vi "Calibration.vi"(0 "Mode":T3, 5 "Calib file":path, 9 "Simulate/Run":T2) -> (14 "Calib const":string[][](array[string]), 16 "Coefficients":dbl[][](array[numeric]) format="%.2f", 19 "Status Out":T1)   [LabVIEW 2010]
uses:
  Anemometry Sub Vis/Calibration/Calib_mode.ctl
  Anemometry Sub Vis/Controls/User_Specific_mode.ctl
  Anemometry Sub Vis/Gen Trav/Multi_Run_Status.ctl
  Anemometry Sub Vis/Controls/Post_Process.ctl
  Anemometry Sub Vis/File/Setup_Filetype.ctl
  Anemometry Sub Vis/Controls/Save_Data.ctl
  Anemometry Sub Vis/Controls/Setup.ctl
  Anemometry Sub Vis/Controls/App_Global.ctl
  Anemometry Sub Vis/Globals/Meas_global.vi
  Anemometry Sub Vis/Globals/Calib_global.vi
  Anemometry Sub Vis/Globals/Plug_in_data_global.vi
  Anemometry Sub Vis/Acquisition/PWA/PWAtasksGLOBAL.vi
  <vilib>/Analysis/NI_AALBase.lvlib
panel:
  in  "-ve Ref Values":bool
  out "String":string
  in  "polynomial order":i32=2 min=1 max=3 step=1
  out "Ref velocity":dbl[](array[numeric])=[2.4275346736, 2.4395664609, 2.453235235, 2.4247395837, 2.4277603784, 2.41169823, 2.4254144559, 2.424896502176921] format="%.3f"
  out "labels":string[](array[string])=["XW1 Volt", "XW2 Volt", "Entered Val", "Selector"]
  in  "Point selector 3":cluster{"Y":dbl, "X":dbl, "t/f":bool}[](array[cluster]) {"X" format="%#.2g"; "Y" format="%#.3f"}
  in  "n":dbl=0.45 format="%.4f"
  in  "Fixed n":bool=TRUE
  out "Sample of input signals":dbl[][](graph)
  in  "Sampling speeds":T4={"Samples /ch"=600, "Sampling Rate /ch (Hz)"=100.0} {"Sampling Rate /ch (Hz)" min=0 format="%.2f"; "Samples /ch" min=0 step=1}
  out "Calibration plot":cluster{cluster{dbl, dbl}[]}[](graph)
  in  "Point selector 4":T5(array[cluster]) {"Y2" format="%#.2f"; "X" format="%#.3f"; "Y" format="%#.2f"}
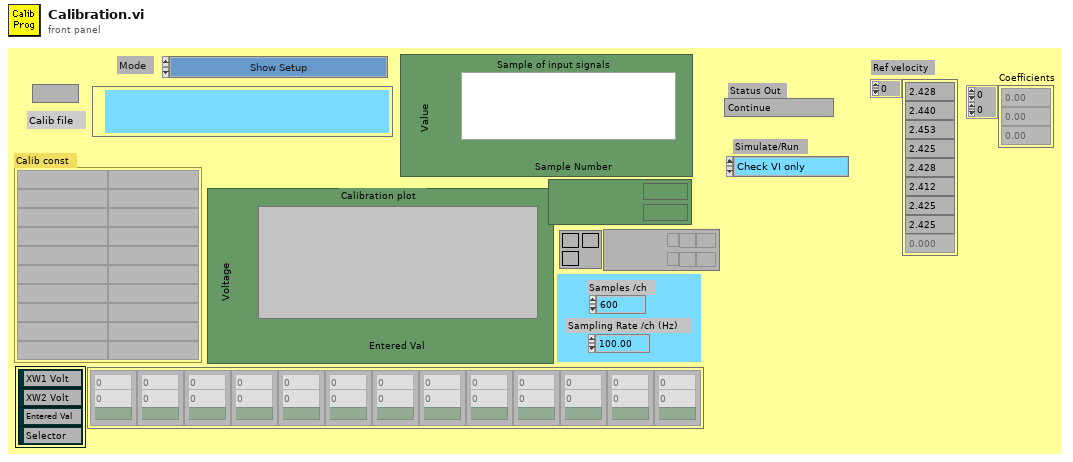
[diagram p1: front panel]
types:
  T1 = typedef "Multi_Run_Status.ctl" = enum16{"Continue", "Jump to Next Point", "Jump to Next Row", "Jump To Fall Back", "Terminate Run"}
  T2 = typedef "User_Specific_mode.ctl" = enum16{"Check VI only", "Run VI"}
  T3 = typedef "Calib_mode.ctl" = enum16{"Show Setup", "Take a New Calibration Point", "Refit Curve", "Setup Front Panel"}
  T4 = cluster{"Samples /ch":i32, "Sampling Rate /ch (Hz)":sgl}
  T5 = cluster{"Y":dbl, "Y2":dbl, "X":dbl, "t/f":bool}[]
  T6 = typedef "Post_Process.ctl" = enum16{"Take New Data", "Post Process Raw Data File"}
  T7 = typedef "Setup_Filetype.ctl" = enum16{"Measurement Setups", "Calibration Setups", "General", "Results File Plotter Setups", "Speed Calib Tweaks"}
  T8 = typedef "Save_Data.ctl" = enum16{"Save No Data", "Save Data"}
  T9 = typedef "Setup.ctl" = enum16{"Run Program", "Show Setup", "Save Current Setup", "Setup Front Panel"}
  T10 = typedef "App_Global.ctl" = enum16{"Read Global", "Write to Global", "Initialise Array"}
  T11 = enum32{"existing file", "new file", "new or existing file", "existing dir", "new dir", "new or existing dir", "existing file (use LLBs)", "new file (use LLBs)", "new or existing file (use LLBs)", "new or existing file or directory (use LLBs)"}
  T12 = typedef "Cal_Inst_type.ctl" = enum16{"Propeller anemometer", "Pressure Transducer", "Hot wire", "Cross wire velocity", "Cross wire angle", "Generic Linear", "Generic Polynomial", "Generic BackPoly", "Fast FID", "Thermocouple", "Cold wire", "Pulsed Wire"}
  T13 = typedef "Ref_Inst_type.ctl" = enum16{"Propellor anemometer", "Pressure Transducer", "Raw voltage", "Pitot-static tube", "Preston tube", "Generic Linear", "Generic Polynomial", "Thermocouple", "LDA", "Enter Value", "ADAM Channel"}
  T14 = cluster{"2nd Ref type":T13, "2nd inst present":bool}
  T15 = typedef "Velocity_cluster.ctl" = cluster{"Name":string, "U":dbl, "u^2":dbl, "u^3/(u^2)^(1.5)":dbl, "u^4/(u^2)^2 -3":dbl, "% u'/U":dbl, "Mean % Err":dbl, "u^4":dbl}
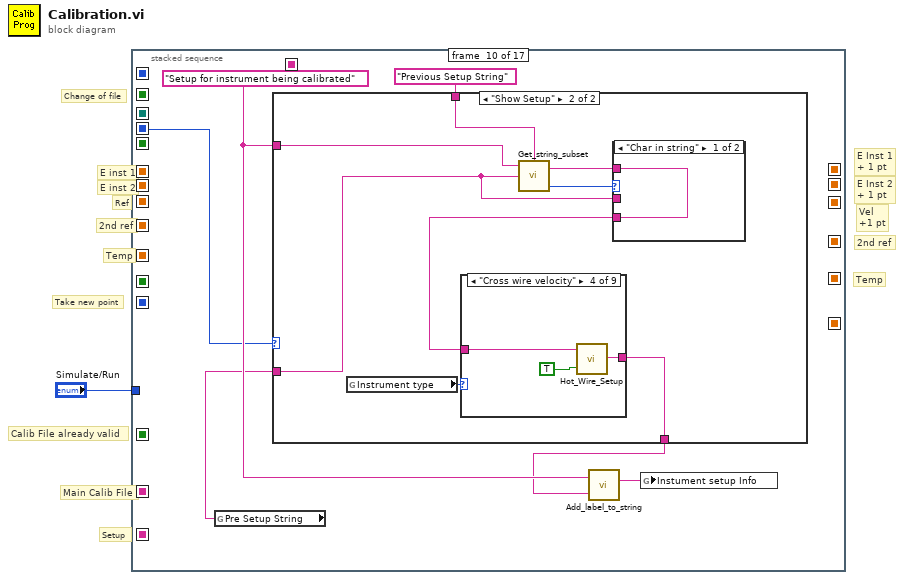
[diagram p0: block diagram]
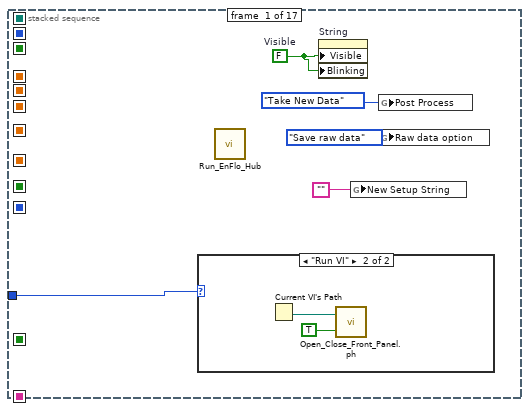
[diagram p2: hidden frame]
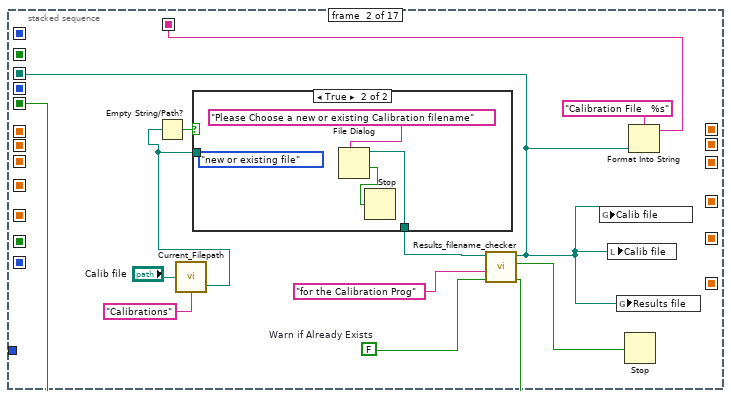
[diagram p4: hidden frame]
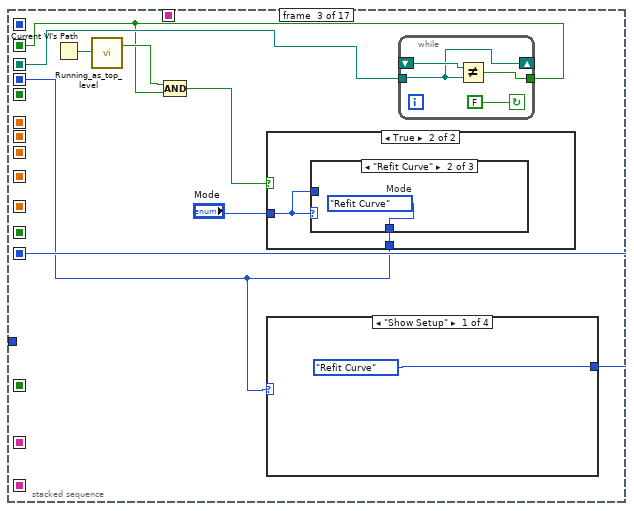
[diagram p6: hidden frame]
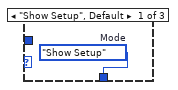
[diagram p8: hidden frame]
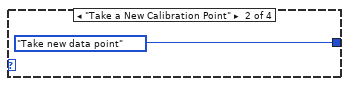
[diagram p10: hidden frame]
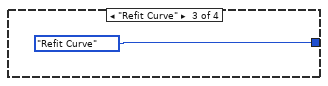
[diagram p11: hidden frame]
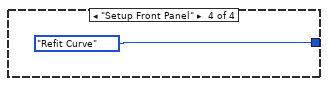
[diagram p12: hidden frame]
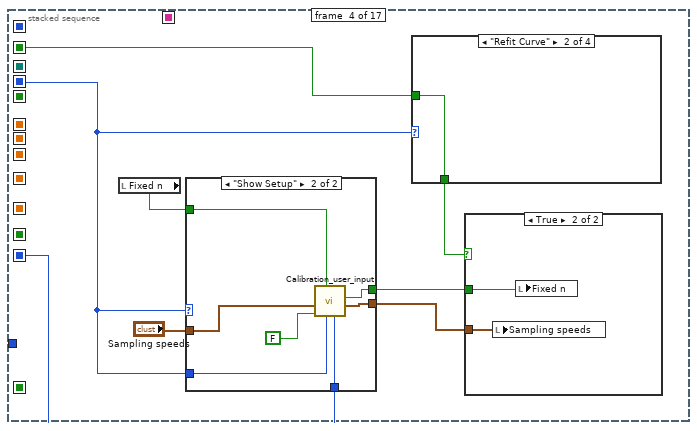
[diagram p13: hidden frame]
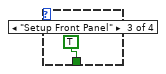
[diagram p15: hidden frame]
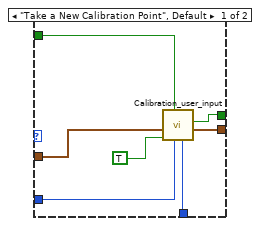
[diagram p18: hidden frame]
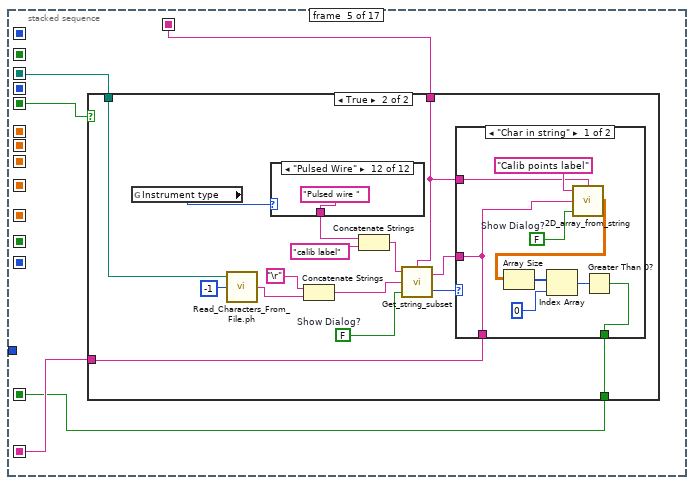
[diagram p19: hidden frame]
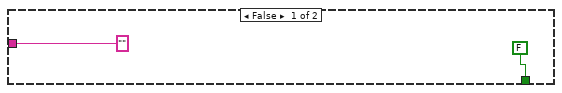
[diagram p20: hidden frame]
diagram:
  # "Change of file"
  # "Take new point"
  # "Calib File already valid"
  # "Main Calib File"
  # "Temp"
  # "Temp"
  # "Setup"
  # "E inst 1"
  # "Ref"
  # "E Inst 1\n+ 1 pt"
  # "Vel\n+1 pt"
  # "E inst 2"
  # "E Inst 2\n+ 1 pt"
  # "2nd ref"
  # "2nd ref"
  n1 = stacked-sequence {
    seq-local: [_ _ _ _ _ _ _ _ _ _ _ w489 _ _ _ _ _] -> [_ _ _ _ _ _ _ _ _ _ _ _ w674 _ _ _ _]
    seq-local: [_ _ _ _ _ _ _ _ _ _ _ w488 _ _ _ _ _] -> [_ _ _ _ _ _ _ _ _ _ _ _ w677 _ _ w740 _]
    seq-local: [_ _ _ _ _ _ _ w376 _ _ _ _ _ _ _ _ _] -> [_ _ _ _ _ _ _ _ _ _ _ w491 _ _ _ _ _]
    seq-local: [_ _ _ _ _ _ _ w375 _ _ _ _ _ _ _ _ _] -> [_ _ _ _ _ _ _ _ _ _ _ w490 _ _ _ _ _]
    seq-local: [_ _ _ _ _ _ _ w374 _ _ _ _ _ _ _ _ _] -> [_ _ _ _ _ _ _ _ _ _ _ w486 _ _ _ _ _]
    seq-local: [_ _ _ _ _ _ _ _ _ _ _ w487 _ _ _ _ _] -> [_ _ _ _ _ _ _ _ _ _ _ _ w676 _ _ _ _]
    seq-local: [_ _ _ _ _ _ _ w373 _ _ _ _ _ _ _ _ _] -> [_ _ _ _ _ _ _ _ _ _ _ w485 _ _ _ _ _]
    seq-local: [_ _ _ _ _ _ _ _ _ _ _ w484 _ _ _ _ _] -> [_ _ _ _ _ _ _ _ _ _ _ _ w671 _ _ _ _]
    seq-local: [_ _ _ _ w78 _ _ _ _ _ _ _ _ _ _ _ _] -> [_ _ _ _ _ _ _ w362 _ _ _ _ _ _ _ _ _]
    seq-local: [_ _ _ _ w79 _ _ _ _ _ _ _ _ _ _ _ _] -> [_ _ _ _ _ _ _ w363 _ _ _ _ _ _ _ _ _]
    seq-local: [_ _ _ _ _ _ _ _ _ _ w464 _ _ _ _ _ _] -> [_ _ _ _ _ _ _ _ _ _ _ _ _ _ w718 _ _]
    seq-local: [_ _ _ _ _ _ _ _ _ _ _ w482 _ _ _ _ _] -> [_ _ _ _ _ _ _ _ _ _ _ _ w675 _ _ _ _]
    seq-local: [_ _ _ _ _ _ _ w372 _ _ _ _ _ _ _ _ _] -> [_ _ _ _ _ _ _ _ _ _ _ w481 _ _ _ _ _]
    seq-local: [_ w13 _ _ _ _ _ _ _ _ _ _ _ _ _ _ _] -> [_ _ w29 _ w77 _ _ _ _ _ w465 w479 _ w700 w727 w741 _]
    seq-local: [_ w18 _ _ _ _ _ _ _ _ _ _ _ _ _ _ _] -> [_ _ _ _ w76 _ _ _ w405 _ _ _ _ _ _ _ _]
    seq-local: [_ _ w32 _ _ _ _ _ _ _ _ _ _ _ _ _ _] -> [_ _ _ w50 _ _ _ _ _ _ _ w478 _ _ _ w742 _]
    seq-local: [_ _ w25 _ _ _ _ _ _ _ _ _ _ _ _ _ _] -> [_ _ _ w49 _ _ _ _ _ w422 _ _ _ _ _ _ w786]
    seq-local: [_ _ _ _ _ _ _ w364 _ _ _ _ _ _ _ _ _] -> [_ _ _ _ _ _ _ _ w403 _ _ _ _ _ _ _ _]
    seq-local: [_ _ _ _ _ _ _ _ _ _ _ _ w672 _ _ _ _] -> [_ _ _ _ _ _ _ _ _ _ _ _ _ w684 _ _ _]
    seq-local: [_ _ _ _ _ _ _ _ _ _ _ _ w670 _ _ _ _] -> [_ _ _ _ _ _ _ _ _ _ _ _ _ w699 _ _ _]
    seq-local: [_ _ w28 _ _ _ _ _ _ _ _ _ _ _ _ _ _] -> [_ _ _ w47 _ _ _ _ w402 _ _ _ _ _ _ _ _]
    seq-local: [_ w12 _ _ _ _ _ _ _ _ _ _ _ _ _ _ _] -> [_ _ _ _ w75 _ _ w357 _ _ _ _ _ _ _ _ _]
    tunnel: "Simulate/Run" -> [w5 _ _ _ _ _ _ _ _ _ _ _ _ _ _ _ _]
    frame #0 {
      w3 = FALSE  # Visible
      n2 = case shown="\"Run VI\"" w5 {
        frame "Check VI only" {
        }
        frame "Run VI" {
          n3 = Current VI's Path() -> (path=w7:path)
          n4 = call "Open_Close_Front_Panel.ph.vi"("Front Panel Window:Open"=TRUE, "VI path"=w7) -> ()  [unwired: 2 out]
        }
      }
      n5 = call "Run_EnFlo_Hub.vi"() -> ()  [unwired: 8 out]
      n6 = property on="String" class="Str"("Visible"=w3, "Blinking"=w3) -> ()  [unwired: 2 in, 2 out]
      n7 = global write "Calib_global.vi" "New Setup String"("") -> ()
      n8 = global write "Meas_global.vi" "Post Process"(Post_Process."Take New Data" ("Post Process")) -> ()
      n9 = global write "Meas_global.vi" "Raw data option"(enum16{"Save raw data", "Raw data not saved"}."Save raw data" ("Raw data option")) -> ()
    }
    frame #1 {
      w19 = FALSE  # Warn if Already Exists
      n10 = call "Current_Filepath.vi"("Filename in"="Calib file", "Data Type"="Calibrations") -> ("Filename Out"=w10:path)  [unwired: 1 out]
      n11 = Empty String/Path?(string/path=w10) -> (empty?=w15:bool)
      n12 = case shown="True" w15 {
        tunnel: w10 -> [w21 _]
        tunnel: [w21 w23] -> w17
        frame False {
        }
        frame True {
          (unwired) T11."new or existing file" ("select mode (2)")
          n13 = File Dialog(7:"Please Choose a new or existing Calibration filename" ("Promp if not found")) -> (1:w22:bool, 3:w23:path)  [unwired: 1 in, 7 out]
          n14 = Stop(stop? (T)=w22) -> ()
        }
      }
      n15 = call "Results_filename_checker.vi"("Warn if Already Exists"=w19, "Comment"="for the Calibration Prog", "Results file"=w17) -> ("exists?"=w18:bool, "cancelled"=w16:bool, "Results file output"=w13:path)  [unwired: 2 in, 1 out]
      n16 = global write "Calib_global.vi" "Calib file"(w13) -> ()
      n17 = local write "Calib file"(w13) -> ()
      n18 = global write "Meas_global.vi" "Results file"(w13) -> ()
      n19 = Stop(stop? (T)=w16) -> ()
      n20 = Format Into String(format string="Calibration File   %s", w13) -> (resulting string=w12:string)  [unwired: 2 in, 1 out]
    }
    frame #2 {
      n21 = Current VI's Path() -> (path=w31:path)
      n22 = call "Running_as_top_level.vi"("Vi path name"=w31) -> ("Top Level"=w30:bool)  [unwired: 1 out]
      n23 = while {
        shift-right: [w41] -> _
        shift-left: _ -> [w42]
        tunnel: w29 -> [w41]
        tunnel: [w40] -> w28
        stop <- FALSE continue-if-true
        n24 = Not Equal?(x=w42, y=w41) -> (x != y?=w40:bool)
      }
      n25 = Compound Arithmetic op=AND(w30, w28) -> (w27:bool)
      n26 = case shown="True" w27 {
        tunnel: "Mode" -> [w33 w34]
        tunnel: [w33 w35] -> w25
        frame False {
        }
        frame True {
          n27 = case shown="\"Refit Curve\"" w34 {
            tunnel: [w36 w37 w38] -> w35
            tunnel: w34 -> [_ _ w38]
            frame "Show Setup", Default {
              w36 = Calib_mode."Show Setup"  # Mode
            }
            frame "Refit Curve" {
              w37 = Calib_mode."Refit Curve"  # Mode
            }
            frame "Setup Front Panel" {
            }
          }
        }
      }
      n28 = case shown="\"Show Setup\"" w25 {
        tunnel: [enum16{"Take new data point", "Refit Curve"}."Refit Curve" ("data mode") enum16{"Take new data point", "Refit Curve"}."Take new data point" ("data mode") enum16{"Take new data point", "Refit Curve"}."Refit Curve" ("data mode") enum16{"Take new data point", "Refit Curve"}."Refit Curve" ("data mode")] -> w32
        frame "Show Setup" {
        }
        frame "Take a New Calibration Point" {
        }
        frame "Refit Curve" {
        }
        frame "Setup Front Panel" {
        }
      }
    }
    frame #3 {
      n29 = local read "Fixed n"() -> (w52:bool)
      n30 = case shown="\"Show Setup\"" w49 {
        tunnel: "Sampling speeds" -> [w67 w74]
        tunnel: w49 -> [w65 w72]
        tunnel: w50 -> [w64 w71]
        tunnel: [w63 w70] -> w53
        tunnel: w52 -> [w61 w69]
        tunnel: [w62 w68] -> w51
        frame "Take a New Calibration Point", Default {
          n31 = call "Calibration_user_input.vi"("data mode"=w64, "Mode"=w65, "Fixed n"=w61, "OK"=TRUE, "Sampling speeds"=w67) -> ("Sampling speeds Output"=w63:T4, "Fixed n out"=w62:bool)  [unwired: 2 in, 3 out]
        }
        frame "Show Setup" {
          n32 = call "Calibration_user_input.vi"("data mode"=w71, "Mode"=w72, "Fixed n"=w69, "OK"=FALSE, "Sampling speeds"=w74) -> ("Sampling speeds Output"=w70:T4, "Fixed n out"=w68:bool)  [unwired: 5 out]
        }
      }
      n33 = case shown="\"Refit Curve\"" w49 {
        tunnel: [w55 w56 TRUE w58] -> w48
        tunnel: w47 -> [w55 w56 _ w58]
        frame "Show Setup" {
        }
        frame "Refit Curve" {
        }
        frame "Setup Front Panel" {
        }
        frame "Take a New Calibration Point" {
        }
      }
      n34 = case shown="True" w48 {
        tunnel: w53 -> [_ w60]
        tunnel: w51 -> [_ w59]
        frame False {
        }
        frame True {
          n35 = local write "Sampling speeds"(w60) -> ()
          n36 = local write "Fixed n"(w59) -> ()
        }
      }
    }
    frame #4 {
      n37 = case shown="True" w76 {
        tunnel: ["" ("Output string") w96] -> w79
        tunnel: [FALSE w95] -> w78
        tunnel: w77 -> [_ w87]
        tunnel: w75 -> [_ w82]
        frame False {
        }
        frame True {
          w86 = FALSE  # Show Dialog?
          n38 = global read "Calib_global.vi" "Instrument type"() -> (w90:T12)
          n39 = call "Read_Characters_From_File.ph.vi"("file path (dialog if empty)"=w87, "number of characters (all:-1)"=-1) -> ("character string"=w84:string)  [unwired: 7 out]
          n40 = case shown="\"Pulsed Wire\"" w90 {
            tunnel: ["Prop " "Mano " "HW " "Cross wire velocity " "Cross wire angle " "Generic Inst " "Generic Polynomial " "Generic BackPoly " "Fast FID " "Thermocouple " "Cold wire " "Pulsed wire "] -> w91
            frame "Propeller anemometer" {
            }
            frame "Pressure Transducer" {
            }
            frame "Hot wire" {
            }
            frame "Cross wire velocity" {
            }
            frame "Cross wire angle" {
            }
            frame "Generic Linear" {
            }
            frame "Generic Polynomial" {
            }
            frame "Generic BackPoly" {
            }
            frame "Fast FID" {
            }
            frame "Thermocouple" {
            }
            frame "Cold wire" {
            }
            frame "Pulsed Wire" {
            }
          }
          n41 = Concatenate Strings("\r", w84) -> (w83:string)
          n42 = Concatenate Strings(w91, "calib label") -> (w92:string)
          n43 = call "Get_string_subset.vi"("String Name"=w82, "Show Dialog?"=w86, "String to split"=w83, "File Label"=w92) -> ("Status"=w89:enum16{"Char in string", "Char not in string"}, "Output string"=w88:string)
          n44 = case shown="\"Char in string\"" w89 {
            tunnel: w88 -> [w115 _]
            tunnel: [w115 ""] -> w96
            tunnel: [w110 FALSE] -> w95
            tunnel: w82 -> [w109 _]
            frame "Char in string" {
              w116 = FALSE  # Show Dialog?
              n45 = call "2D_array_from_string.vi"("String Name"=w109, "Show Dialog?"=w116, "Input string"=w115, "Array title"="Calib points label") -> ("2D data array"=w114:dbl[][])
              n46 = Array Size(array=w114) -> (size(s)=w113:i32[])
              n47 = Index Array(array=w113, index=0 ("Index")) -> (element=w111:i32)
              n48 = Greater Than 0?(x=w111) -> (x > 0?=w110:bool)
            }
            frame "Char not in string" {
            }
          }
        }
      }
    }
    frame #5 {
      w122 = ""
      n49 = global read "Calib_global.vi" "2nd ref instrument"() -> (w129:T14)
      n50 = global read "Calib_global.vi" "Ref Instrument type"() -> (w130:T13)
      n51 = Unbundle By Name(w129) -> ("2nd Ref type"=w127:T13, "2nd inst present"=w128:bool)
      n52 = global read "Calib_global.vi" "Instrument type"() -> (w133:T12)
      n53 = case shown="\"Propellor anemometer\"" w130 {
        tunnel: [w159 w162 w166 w168 w171 w174 w177 w180 w183 string[] [] string[] []] -> w126
        tunnel: [FALSE FALSE FALSE FALSE TRUE FALSE FALSE FALSE FALSE FALSE FALSE] -> w121
        frame "Propellor anemometer" {
          n54 = Build Array("Prop Velocity") -> (w159:string[])
        }
        frame "Pressure Transducer" {
          n55 = Build Array("Pressure Trans") -> (w162:string[])
        }
        frame "Raw voltage" {
          n56 = Build Array("Raw Voltage") -> (w166:string[])
        }
        frame "Pitot-static tube" {
          n57 = Build Array("Pitot Vel") -> (w168:string[])
        }
        frame "Preston tube" {
          n58 = Build Array("Shear stress") -> (w171:string[])
        }
        frame "Generic Linear" {
          n59 = Build Array("Gen Lin") -> (w174:string[])
        }
        frame "Generic Polynomial" {
          n60 = Build Array("Gen Poly") -> (w177:string[])
        }
        frame "Thermocouple" {
          n61 = Build Array("Thermo") -> (w180:string[])
        }
        frame "LDA" {
          n62 = Build Array("LDA Vel") -> (w183:string[])
        }
        frame "Enter Value" {
        }
        frame "ADAM Channel" {
        }
      }
      n63 = case shown="True" w128 {
        tunnel: w127 -> [_ w136]
        tunnel: [w135 w137] -> w124
        tunnel: w126 -> [w135 _]
        frame False {
        }
        frame True {
          n64 = case shown="\"Propellor anemometer\"" w136 {
            tunnel: [w138 w140 w143 w144 w146 w148 w150 w152 w154 string[] [] string[] []] -> w137
            frame "Propellor anemometer" {
              n65 = Build Array("Prop Velocity") -> (w138:string[])
            }
            frame "Pressure Transducer" {
              n66 = Build Array("Pressure Trans") -> (w140:string[])
            }
            frame "Raw voltage" {
              n67 = Build Array("Raw Voltage") -> (w143:string[])
            }
            frame "Pitot-static tube" {
              n68 = Build Array("Pitot Vel") -> (w144:string[])
            }
            frame "Preston tube" {
              n69 = Build Array("Shear stress") -> (w146:string[])
            }
            frame "Generic Linear" {
              n70 = Build Array("Gen Lin") -> (w148:string[])
            }
            frame "Generic Polynomial" {
              n71 = Build Array("Gen Poly") -> (w150:string[])
            }
            frame "Thermocouple" {
              n72 = Build Array("Thermo") -> (w152:string[])
            }
            frame "LDA" {
              n73 = Build Array("LDA Vel") -> (w154:string[])
            }
            frame "Enter Value" {
            }
            frame "ADAM Channel" {
            }
          }
        }
      }
      n74 = case shown="\"Pulsed Wire\"" w133 {
        tunnel: [w193 w197 w201 w205 w210 w215 w219 w223 w227 w231 w235 w240] -> w123
        tunnel: [FALSE FALSE FALSE FALSE FALSE FALSE TRUE TRUE FALSE FALSE TRUE TRUE] -> w125
        tunnel: [w191 w195 w199 w203 w208 w213 w217 w221 w225 w229 w233 FALSE] -> w120
        tunnel: w121 -> [w191 w195 w199 w203 w208 w213 w217 w221 w225 w229 w233 _]
        frame "Propeller anemometer" {
          n75 = Build Array("Prop Voltage") -> (w193:string[])
        }
        frame "Pressure Transducer" {
          n76 = Build Array("Pressure Trans") -> (w197:string[])
        }
        frame "Hot wire" {
          n77 = Build Array("HW Voltage") -> (w201:string[])
        }
        frame "Cross wire velocity" {
          n78 = Build Array("XW1 Voltage", "XW2 Voltage") -> (w205:string[])
        }
        frame "Cross wire angle" {
          n79 = Build Array("XW1 Voltage", "XW2 Voltage") -> (w210:string[])
        }
        frame "Generic Linear" {
          n80 = Build Array("Generic Voltage") -> (w215:string[])
        }
        frame "Generic Polynomial" {
          n81 = Build Array("Generic Voltage") -> (w219:string[])
        }
        frame "Generic BackPoly" {
          n82 = Build Array("Generic Voltage") -> (w223:string[])
        }
        frame "Fast FID" {
          n83 = Build Array("FF Voltage") -> (w227:string[])
        }
        frame "Thermocouple" {
          n84 = Build Array("Thermo Voltage") -> (w231:string[])
        }
        frame "Cold wire" {
          n85 = Build Array("CW Voltage") -> (w235:string[])
        }
        frame "Pulsed Wire" {
          n86 = local write "polynomial order"(3 ("polynomial order")) -> ()
          n87 = Build Array("PWA 1/TOF") -> (w240:string[])
        }
      }
      n88 = property on="polynomial order" class="DigNum (strict)"("Visible"=w125) -> ()  [unwired: 2 in, 2 out]
      n89 = Build Array (concatenate)(w124, w123, w122, w122, w122) -> (w131:string[])
      n90 = for {
        N: 3 -> [_]
        tunnel: w131 -> [w189] mode=indexing
        i -> [w190]
        n91 = property on="Sample of input signals" class="WFGraph (strict)"("Active Plot"=w190, "Plot.Plot Name"=w189) -> ()  [unwired: 2 in, 2 out]
      }
      n92 = case shown="False" w120 {
        frame False {
          n93 = local write "-ve Ref Values"(FALSE ("-ve Ref Values")) -> ()
        }
        frame True {
        }
      }
      n94 = property on="-ve Ref Values" class="Bool (strict)"("Visible"=w120) -> ()  [unwired: 2 in, 2 out]
    }
    frame #6 {
      n95 = global read "Calib_global.vi" "Instrument type"() -> (w245:T12)
      n96 = global read "Calib_global.vi" "Ref Instrument type"() -> (w244:T13)
      n97 = case shown="\"Propellor anemometer\"" w244 {
        tunnel: ["Prop Vel" "Pressure" "Voltage" "Pitot Vel" "Shear stress" "Generic Linear" "Generic Poly" "Thermo T" "LDA Vel" "Entered Val" "ADAM Channel"] -> w247
        frame "Propellor anemometer" {
        }
        frame "Pressure Transducer" {
        }
        frame "Raw voltage" {
        }
        frame "Pitot-static tube" {
        }
        frame "Preston tube" {
        }
        frame "Generic Linear" {
        }
        frame "Generic Polynomial" {
        }
        frame "Thermocouple" {
        }
        frame "LDA" {
        }
        frame "Enter Value" {
        }
        frame "ADAM Channel" {
        }
      }
      n98 = case shown="\"Pulsed Wire\"" w245 {
        tunnel: [FALSE FALSE TRUE TRUE TRUE FALSE FALSE FALSE FALSE FALSE FALSE FALSE] -> w250
        tunnel: [TRUE TRUE TRUE FALSE FALSE TRUE TRUE TRUE TRUE TRUE TRUE TRUE] -> w249
        tunnel: [FALSE FALSE FALSE TRUE TRUE FALSE FALSE FALSE FALSE FALSE FALSE FALSE] -> w248
        tunnel: w247 -> [w263 w270 w279 w289 w299 w309 w315 w322 w329 w337 w343 w350]
        tunnel: [w266 w273 w282 w292 w302 w311 w318 w325 w332 w339 w346 w353] -> w246
        tunnel: "Selector" -> [w265 w272 w281 w291 w301 w308 w317 w324 w331 w336 w345 w352]
        tunnel: [w264 w271 "E^2" "XW Volt^2" "Y" w310 w315 w323 w329 w338 w343 w350] -> w242
        tunnel: [w263 w270 w277 w287 "X" w309 w316 w322 w330 w337 w344 w351] -> w243
        frame "Propeller anemometer" {
          w264 = "Prop Volt"
          n99 = Build Array(w264, w263, w265) -> (w266:string[])
        }
        frame "Pressure Transducer" {
          w271 = "Voltage"
          n100 = Build Array(w271, w270, w272) -> (w273:string[])
        }
        frame "Hot wire" {
          n101 = Build Array("HW Volt", w279, w281) -> (w282:string[])
          n102 = Concatenate Strings(w279, "^n") -> (w277:string)
        }
        frame "Cross wire velocity" {
          n103 = Build Array("XW1 Volt", "XW2 Volt", w289, w291) -> (w292:string[])
          n104 = Concatenate Strings(w289, "^n") -> (w287:string)
        }
        frame "Cross wire angle" {
          n105 = Build Array("XW1 Volt", "XW2 Volt", w299, w301) -> (w302:string[])
        }
        frame "Generic Linear" {
          w310 = "Gen Volt"
          n106 = Build Array(w310, w309, w308) -> (w311:string[])
        }
        frame "Generic Polynomial" {
          w316 = "Gen Volt"
          n107 = Build Array(w316, w315, w317) -> (w318:string[])
        }
        frame "Generic BackPoly" {
          w323 = "Gen Volt"
          n108 = Build Array(w322, w323, w324) -> (w325:string[])
        }
        frame "Fast FID" {
          w330 = "FF Volt"
          n109 = Build Array(w330, w329, w331) -> (w332:string[])
        }
        frame "Thermocouple" {
          w338 = "Thermo Volt"
          n110 = Build Array(w338, w337, w336) -> (w339:string[])
        }
        frame "Cold wire" {
          w344 = "CW Volt"
          n111 = Build Array(w344, w343, w345) -> (w346:string[])
        }
        frame "Pulsed Wire" {
          w351 = "1/TOF"
          n112 = Build Array(w351, w350, w352) -> (w353:string[])
        }
      }
      "labels" <- w246
      n113 = property on="n" class="DigNum (strict)"("Visible"=w250) -> ()  [unwired: 2 in, 2 out]
      n114 = property on="Fixed n" class="Bool (strict)"("Visible"=w250) -> ()  [unwired: 2 in, 2 out]
      n115 = property on="Calibration plot" class="XYGraph (strict)"("X Scale.Name Label.Text"=w243, "Y Scale.Name Label.Text"=w242) -> ()  [unwired: 2 in, 2 out]
      n116 = property on="Point selector 3" class="Arr (strict)"("Visible"=w249) -> ()  [unwired: 2 in, 2 out]
      n117 = property on="Point selector 4" class="Arr (strict)"("Visible"=w248) -> ()  [unwired: 2 in, 2 out]
    }
    frame #7 {
      # "Case structure to read previous calibration points if required"
      n118 = global read "Calib_global.vi" "Calibration Points"() -> (w361:dbl[])
      n119 = case shown="True" w362 {
        tunnel: w363 -> [_ w396]
        tunnel: [w388 w393] -> w360
        tunnel: w361 -> [w389 w392]
        tunnel: w357 -> [_ w390]
        frame False {
          n120 = Build Array(w389) -> (w388:dbl[][])
        }
        frame True {
          w395 = FALSE  # Show Dialog?
          n121 = Array Size(array=w392) -> (size(s)=w391:i32)
          n122 = call "2D_array_from_string.vi"("String Name"=w390, "Show Dialog?"=w395, "Input string"=w396, "Array title"="Calib points label") -> ("2D data array"=w394:dbl[][])
          n123 = case shown="0" w391 {
            tunnel: w394 -> [w398 w401]
            tunnel: [w398 w400] -> w393
            tunnel: w392 -> [_ w399]
            frame 0 {
            }
            frame 1, Default {
              n124 = Build Array (concatenate)(w401, w399) -> (w400:dbl[][])
            }
          }
        }
      }
      n125 = for {
        tunnel: w360 -> [w378] mode=indexing
        shift-right: [w377] -> w358
        shift-left: dbl[][] [] -> [w379]
        n126 = Array Subset(array=w378, length=2) -> (w382:dbl[])  [unwired: 1 in]
        n127 = Not A Number/Path/Refnum?(number/path/refnum=w382) -> (NaN/Path/Refnum?=w381:bool[])
        n128 = Or Array Elements(Boolean array=w381) -> (logical OR=w380:bool)
        n129 = case shown="False" w380 {
          tunnel: w379 -> [w386 w387]
          tunnel: w378 -> [w385 _]
          tunnel: [w384 w387] -> w377
          frame False {
            n130 = Build Array (concatenate)(w386, w385) -> (w384:dbl[][])
          }
          frame True {
          }
        }
      }
      n131 = Index Array(array=w358, index (col)=0) -> (element=w375:dbl[])  [unwired: 1 in]
      n132 = Index Array(array=w358, index (col)=1) -> (element=w376:dbl[])  [unwired: 1 in]
      n133 = Index Array(array=w358, index (col)=2) -> (element=w374:dbl[])  [unwired: 1 in]
      n134 = Index Array(array=w358, index (col)=3) -> (element=w373:dbl[])  [unwired: 1 in]
      n135 = Index Array(array=w358, index (col)=4) -> (element=w372:dbl[])  [unwired: 1 in]
      n136 = Index Array(array=w358, index (col)=5) -> (element=w365:dbl[])  [unwired: 1 in]
      n137 = Not A Number/Path/Refnum?(number/path/refnum=w365) -> (NaN/Path/Refnum?=w364:bool[])
    }
    frame #8 {
      n138 = And(x=w402, y=w405) -> (x .and. y?=w404:bool)
      n139 = case shown="True" w404 {
        tunnel: w403 -> [_ w406]
        frame False {
        }
        frame True {
          n140 = local read "Point selector 3"() -> (w410:cluster{"Y":dbl, "X":dbl, "t/f":bool}[])
          n141 = local read "Point selector 4"() -> (w407:T5)
          n142 = for {
            tunnel: w410 -> [w418]
            tunnel: [w420] -> w409 mode=indexing
            tunnel: w406 -> [w419] mode=indexing
            i -> [w417]
            n143 = Index Array(array=w418, index=w417) -> (element=w416:cluster{"Y":dbl, "X":dbl, "t/f":bool})
            n144 = Bundle By Name(cluster=w416, "t/f"=w419) -> (w420:cluster{"Y":dbl, "X":dbl, "t/f":bool})
          }
          n145 = for {
            tunnel: w407 -> [w413]
            tunnel: [w415] -> w408 mode=indexing
            tunnel: w406 -> [w414] mode=indexing
            i -> [w412]
            n146 = Index Array(array=w413, index=w412) -> (element=w411:cluster{"Y":dbl, "Y2":dbl, "X":dbl, "t/f":bool})
            n147 = Bundle By Name(cluster=w411, "t/f"=w414) -> (w415:cluster{"Y":dbl, "Y2":dbl, "X":dbl, "t/f":bool})
          }
          n148 = local write "Point selector 3"(w409) -> ()
          n149 = local write "Point selector 4"(w408) -> ()
        }
      }
    }
    frame #9 {
      w425 = "Setup for instrument being calibrated"
      n150 = global read "Calib_global.vi" "Pre Setup String"() -> (w423:string)
      n151 = case shown="\"Show Setup\"" w422 {
        tunnel: w423 -> [w430 w434]
        tunnel: w425 -> [w429 w433]
        tunnel: [w428 w432] -> w424
        tunnel: "Previous Setup String" ("String Name") -> [w427 w431]
        frame "Take a New Calibration Point", Default {
          n152 = call "Get_string_subset.vi"("String Name"=w427, "String to split"=w430, "File Label"=w429) -> ("Output string"=w428:string)  [unwired: 1 in, 1 out]
        }
        frame "Show Setup" {
          n153 = global read "Calib_global.vi" "Instrument type"() -> (w438:T12)
          n154 = call "Get_string_subset.vi"("String Name"=w431, "String to split"=w434, "File Label"=w433) -> ("Status"=w436:enum16{"Char in string", "Char not in string"}, "Output string"=w437:string)  [unwired: 1 in]
          n155 = case shown="\"Char in string\"" w436 {
            tunnel: [w439 w440] -> w435
            tunnel: w437 -> [w439 _]
            tunnel: w434 -> [_ w440]
            frame "Char in string" {
            }
            frame "Char not in string" {
            }
          }
          n156 = case shown="\"Cross wire velocity\"" w438 {
            tunnel: [w442 w444 w447 w450 w453 w455 w457 w459 ""] -> w432
            tunnel: w435 -> [w441 w443 w445 w448 w451 w454 w456 w458 _]
            frame "Propeller anemometer" {
              n157 = call "Propeller_setup.vi"("Setup String"=w441) -> ("Output string"=w442:string)
            }
            frame "Pressure Transducer" {
              n158 = call "Pressure_Transducer_Setup.vi"("Setup String"=w443) -> ("Output string"=w444:string)
            }
            frame "Hot wire" {
              n159 = call "Hot_Wire_Setup.vi"("XW?"=FALSE, "Setup String"=w445) -> ("Output string"=w447:string)
            }
            frame "Cross wire velocity" {
              n160 = call "Hot_Wire_Setup.vi"("XW?"=TRUE, "Setup String"=w448) -> ("Output string"=w450:string)
            }
            frame "Cross wire angle" {
              n161 = call "Hot_Wire_Setup.vi"("XW?"=TRUE, "Setup String"=w451) -> ("Output string"=w453:string)
            }
            frame "Generic Linear" {
              n162 = call "Generic_setup.vi"("Setup String"=w454) -> ("Output String"=w455:string)
            }
            frame "Generic Polynomial" {
              n163 = call "Generic_setup.vi"("Setup String"=w456) -> ("Output String"=w457:string)
            }
            frame "Generic BackPoly" {
              n164 = call "Generic_setup.vi"("Setup String"=w458) -> ("Output String"=w459:string)
            }
            frame "Fast FID", Default {
            }
          }
        }
      }
      n165 = call "Add_label_to_string.vi"("String to write"=w424, "File Label"=w425) -> ("Output string"=w426:string)
      n166 = global write "Calib_global.vi" "Instument setup Info"(w426) -> ()
    }
    frame #10 {
      w466 = TRUE  # Lock File
      w472 = FALSE  # advisory dialog? (display:T)
      w473 = FALSE  # append to file? (new file:F)
      n167 = global read "Calib_global.vi" "Instument setup Info"() -> (w468:string)
      n168 = Path To String(path=w465) -> (string=w467:string)
      n169 = global read "Calib_global.vi" "New Setup String"() -> (w469:string)
      n170 = call "Date_and_Time_to_string.vi"() -> ("Date and time (spreadsheet)"=w475:string)
      n171 = call "Characters_to_string.vi"("Characters to write"=w467, "Label for characters"="Calib filename") -> ("Output string"=w476:string)
      n172 = Concatenate Strings(w475, w476, w469, w468) -> (w464:string)
      n173 = call "Add_label_to_string.vi"("String to write"=w464, "File Label"="Raw data header") -> ("Output string"=w470:string)
      n174 = call "Setup_Filepath.vi"("Setup File Type"=Setup_Filetype."Calibration Setups", "Filename in"="Current_Setup.xls") -> ("Filename Out"=w461:path)  [unwired: 1 out]
      n175 = call "Calib_read_files.vi"() -> ()  [unwired: 1 out]
      n176 = call "Write_Characters_To_File.vi"("file path (dialog if empty)"=w461, "advisory dialog? (display:T)"=w472, "character string"=w470, "append to file? (new file:F)"=w473, "Lock File"=w466) -> ()  [unwired: 4 out]
    }
    frame #11 {
      # "Case structure for the decision 'MORE POINTS' or 'REFIT CURVE'"
      n177 = global read "Calib_global.vi" "2nd ref instrument"() -> (w483:T14)
      n178 = global read "Calib_global.vi" "Instrument type"() -> (w477:T12)
      n179 = case shown="\"Take new data point\"" w478 {
        tunnel: [w502 w669] -> w488
        tunnel: [w503 w665] -> w489
        tunnel: w491 -> [w504 w669]
        tunnel: w490 -> [w505 w665]
        tunnel: [w501 w668] -> w487
        tunnel: w486 -> [w500 w668]
        tunnel: w485 -> [w499 w667]
        tunnel: [w497 w667] -> w484
        tunnel: w483 -> [w498 _]
        tunnel: [w495 w666] -> w482
        tunnel: w481 -> [w496 w666]
        tunnel: w479 -> [w494 _]
        tunnel: [w493 Multi_Run_Status."Continue" ("Status Out")] -> w480
        tunnel: w477 -> [w492 _]
        frame "Take new data point" {
          # "Start"
          # "Taking data for another calibration point"
          n180 = stacked-sequence {
            seq-local: [_ _ _ _ w557 _ _ _] -> [_ _ _ _ _ w577 _ _]
            seq-local: [w509 _ _ _ _ _ _ _] -> [_ _ _ _ w559 w570 _ _]
            seq-local: [_ _ w533 _ _ _ _ _] -> [_ _ _ _ w558 w569 w602 _]
            seq-local: [_ _ _ _ _ w568 _ _] -> [_ _ _ _ _ _ w601 _]
            seq-local: [_ _ w532 _ _ _ _ _] -> [_ _ _ _ _ w567 w600 _]
            seq-local: [_ _ _ w538 _ _ _ _] -> [_ _ _ _ w553 _ _ _]
            seq-local: [_ _ _ w536 _ _ _ _] -> [_ _ _ _ _ _ w598 _]
            seq-local: [_ _ _ w535 _ _ _ _] -> [_ _ _ _ _ _ w597 _]
            seq-local: [_ _ _ w534 _ _ _ _] -> [_ _ _ _ _ w565 _ _]
            tunnel: w504 -> [_ _ _ _ _ _ w606 _]
            tunnel: [_ _ _ _ w561 _ _ _] -> w503
            tunnel: w505 -> [_ _ _ _ w560 _ _ _]
            tunnel: [_ _ _ _ _ _ w605 _] -> w502
            tunnel: [_ _ _ _ _ _ w604 _] -> w501
            tunnel: w500 -> [_ _ _ _ _ _ w603 _]
            tunnel: w499 -> [_ _ _ _ _ w573 _ _]
            tunnel: [_ _ _ _ _ w572 _ _] -> w497
            tunnel: w498 -> [_ _ _ _ _ w571 _ _]
            tunnel: w496 -> [_ w514 _ _ _ _ _ _]
            tunnel: [_ w513 _ _ _ _ _ _] -> w495
            tunnel: w494 -> [_ w511 _ _ _ _ _ _]
            tunnel: [_ w512 _ _ _ _ _ _] -> w493
            tunnel: w492 -> [_ _ _ w537 _ w566 w599 _]
            frame #0 {
              w506 = TRUE  # Visible
              w507 = "Current Taking a New Calibration Point"  # String
              n181 = Get Date/Time In Seconds() -> (seconds since 1Jan1904=w508:timestamp)
              n182 = To Double Precision Float(number=w508) -> (double precision float=w509:dbl)
              n183 = property on="String" class="Str"("Visible"=w506, "Blinking"=w506) -> ()  [unwired: 2 in, 2 out]
              "String" <- w507
            }
            frame #1 {
              # "Acquire data from input channels"
              n184 = global read "Calib_global.vi" "Temp (deg C)"() -> (w510:dbl)
              n185 = while {
                tunnel: [w517] -> w512
                tunnel: w511 -> [w516]
                stop <- w515 continue-if-true
                n186 = stacked-sequence {
                  seq-local: [_ w519 _] -> [_ _ w527]
                  tunnel: [_ w519 _] -> w517
                  tunnel: w516 -> [_ w523 _]
                  tunnel: [_ _ w528] -> w515
                  frame #0 {
                    n187 = global write "Meas_global.vi" "Remote control"(TRUE ("Remote control")) -> ()
                  }
                  frame #1 {
                    n188 = call "Get_Data_Base_file_code.vi"("Results Filename"=w523, "Data Type"="Raw_Calibrations") -> ("Raw Data File Name"=w520:path)  [unwired: 3 out]
                    n189 = call "Measurement.vi"("setup"=Setup."Run Program", "Post Process"=Post_Process."Take New Data", "File"=Save_Data."Save No Data", "Raw data file"=w520, "Setup filename"="Calib_Setup.xls") -> ("Status Out"=w519:T1)  [unwired: 2 in, 12 out]
                  }
                  frame #2 {
                    n190 = global read "Meas_global.vi" "Repeat Measurement?"() -> (w529:bool)
                    n191 = Equal?(x=w527, y=Multi_Run_Status."Continue" ("Status Out")) -> (x = y?=w530:bool)
                    n192 = And(x=w530, y=w529) -> (x .and. y?=w528:bool)
                  }
                }
              }
              n193 = Build Array (concatenate)(w514, w510) -> (w513:dbl[])
            }
            frame #2 {
              n194 = global read "Plug_in_data_global.vi" "Equi Spaced"() -> (w532:dbl[][])
              "Sample of input signals" <- w532
              n195 = global read "Meas_global.vi" "Velocity Cluster Array"() -> (w533:T15[])
            }
            frame #3 {
              n196 = case shown="\"Propeller anemometer\", Default" w537 {
                tunnel: [0 ("Index in") 1 ("Index in")] -> w538
                tunnel: [w539 w542] -> w536
                tunnel: [w539 w546] -> w535
                tunnel: [w539 w545] -> w534
                frame "Propeller anemometer", Default {
                  w539 = 0.0 ("mean")
                }
                frame "Pulsed Wire" {
                  n197 = global read "PWAtasksGLOBAL.vi" "PWA 1/TOF"() -> (w549:dbl[][])
                  n198 = Index Array(array=w549, index (row)=0) -> (element=w547:dbl[])  [unwired: 1 in]
                  n199 = call "Mean_fr_NaN_data.vi"("Data"=w547) -> ("Mean value"=w542:dbl)
                  n200 = Less Than 0?(x=w542) -> (x < 0?=w541:bool)
                  n201 = local write "-ve Ref Values"(w541) -> ()
                  n202 = Multiply(x=w547, y=w547) -> (x*y=w544:dbl[])
                  n203 = call "Mean_fr_NaN_data.vi"("Data"=w544) -> ("Mean value"=w546:dbl)
                  n204 = Multiply(x=w547, y=w544) -> (x*y=w543:dbl[])
                  n205 = call "Mean_fr_NaN_data.vi"("Data"=w543) -> ("Mean value"=w545:dbl)
                }
              }
            }
            frame #4 {
              # "Adding the velocity value to the array"
              n206 = global read "Calib_global.vi" "ADAM Channel Name"() -> (w551:string)
              n207 = global read "Calib_global.vi" "Ref Instrument type"() -> (w556:T13)
              n208 = call "Get_ref_inst_value.vi"("Ref Instrument type"=w556, "ADAM Channel Name"=w551, "Index in"=w553, "Velocity Cluster Array"=w558, "Start time"=w559) -> ("Ref Value"=w555:dbl, "Index out"=w557:i32)  [unwired: 2 in, 7 out]
              n209 = case shown="True" "-ve Ref Values" {
                tunnel: w555 -> [w562 w564]
                tunnel: [w562 w563] -> w554
                frame False {
                }
                frame True {
                  n210 = Negate(x=w564) -> (-x=w563:dbl)
                }
              }
              n211 = Build Array (concatenate)(w560, w554) -> (w561:dbl[])
            }
            frame #5 {
              n212 = Unbundle(w571) -> ("2nd Ref type"=w575:T13, "2nd inst present"=w574:bool)
              n213 = case shown="True" w574 {
                tunnel: w577 -> [w582 w592]
                tunnel: [w580 w594] -> w576
                tunnel: w575 -> [_ w595]
                tunnel: w570 -> [_ w596]
                tunnel: w569 -> [_ w593]
                tunnel: [w582 w591] -> w568
                tunnel: w567 -> [w581 _]
                tunnel: w566 -> [w579 _]
                tunnel: w565 -> [w578 _]
                frame False {
                  n214 = case shown="\"Propeller anemometer\", Default" w579 {
                    tunnel: w582 -> [_ w588 _]
                    tunnel: w581 -> [_ w587 _]
                    tunnel: [0.0 ("mean") w584 w589] -> w580
                    tunnel: w578 -> [_ _ w589]
                    frame "Propeller anemometer", Default {
                    }
                    frame "Generic Polynomial" {
                      n215 = Index Array(array=w587, index (row)=w588) -> (element=w586:dbl[])  [unwired: 1 in]
                      n216 = Compound Arithmetic op=MULTIPLY(w586, w586, w586) -> (w585:dbl[])
                      n217 = call <vilib>:"Mean.vi"("X"=w585) -> ("mean"=w584:dbl)  [unwired: 1 out]
                    }
                    frame "Pulsed Wire" {
                    }
                  }
                }
                frame True {
                  n218 = global read "Calib_global.vi" "ADAM Channel Name Vel Ref"() -> (w590:string)
                  n219 = call "Get_ref_inst_value.vi"("Ref Instrument type"=w595, "ADAM Channel Name"=w590, "Index in"=w592, "Velocity Cluster Array"=w593, "Start time"=w596) -> ("Ref Value"=w594:dbl, "Index out"=w591:i32)  [unwired: 3 in, 6 out]
                }
              }
              n220 = Build Array (concatenate)(w573, w576) -> (w572:dbl[])
            }
            frame #6 {
              n221 = case shown="\"Pulsed Wire\"" w599 {
                tunnel: w606 -> [w611 w621 w628 w636 w648 w659]
                tunnel: [w612 w622 w629 w637 w649 w660] -> w605
                tunnel: w603 -> [w610 w620 w627 w632 w647 w658]
                tunnel: [w610 w619 w626 w630 w646 w657] -> w604
                tunnel: w602 -> [w608 _ _ w634 w642 w653]
                tunnel: w601 -> [w613 w623 _ w638 w640 w651]
                tunnel: w600 -> [_ w618 _ _ _ _]
                tunnel: w598 -> [_ _ w625 _ _ _]
                tunnel: w597 -> [_ _ w624 _ _ _]
                frame "Propeller anemometer", Default {
                  n222 = Index Array(array=w608, index=w613) -> (element=w609:T15)
                  n223 = Unbundle By Name(w609) -> ("U"=w607:dbl)
                  n224 = Build Array (concatenate)(w611, w607) -> (w612:dbl[])
                }
                frame "Generic Polynomial" {
                  n225 = Index Array(array=w618, index (row)=w623) -> (element=w615:dbl[])  [unwired: 1 in]
                  n226 = call <vilib>:"Mean.vi"("X"=w615) -> ("mean"=w617:dbl)  [unwired: 1 out]
                  n227 = Multiply(x=w615, y=w615) -> (x*y=w614:dbl[])
                  n228 = call <vilib>:"Mean.vi"("X"=w614) -> ("mean"=w616:dbl)  [unwired: 1 out]
                  n229 = Build Array (concatenate)(w621, w617) -> (w622:dbl[])
                  n230 = Build Array (concatenate)(w620, w616) -> (w619:dbl[])
                }
                frame "Pulsed Wire" {
                  n231 = Build Array (concatenate)(w628, w625) -> (w629:dbl[])
                  n232 = Build Array (concatenate)(w627, w624) -> (w626:dbl[])
                }
                frame "Fast FID" {
                  n233 = Index Array(array=w634, index=w638) -> (element=w635:T15)
                  n234 = Unbundle By Name(w635) -> ("U"=w633:dbl, "u^2"=w631:dbl)
                  n235 = Build Array (concatenate)(w636, w633) -> (w637:dbl[])
                  n236 = Build Array (concatenate)(w632, w631) -> (w630:dbl[])
                }
                frame "Cross wire velocity" {
                  n237 = Increment(x=w640) -> (x+1=w639:i32)
                  n238 = Index Array(array=w642, index=w640) -> (element=w645:T15)
                  n239 = Index Array(array=w642, index=w639) -> (element=w644:T15)
                  n240 = Unbundle By Name(w645) -> ("U"=w641:dbl)
                  n241 = Unbundle By Name(w644) -> ("U"=w643:dbl)
                  n242 = Build Array (concatenate)(w648, w641) -> (w649:dbl[])
                  n243 = Build Array (concatenate)(w647, w643) -> (w646:dbl[])
                }
                frame "Cross wire angle" {
                  n244 = Increment(x=w651) -> (x+1=w650:i32)
                  n245 = Index Array(array=w653, index=w651) -> (element=w656:T15)
                  n246 = Index Array(array=w653, index=w650) -> (element=w655:T15)
                  n247 = Unbundle By Name(w656) -> ("U"=w652:dbl)
                  n248 = Unbundle By Name(w655) -> ("U"=w654:dbl)
                  n249 = Build Array (concatenate)(w659, w652) -> (w660:dbl[])
                  n250 = Build Array (concatenate)(w658, w654) -> (w657:dbl[])
                }
              }
            }
            frame #7 {
              w661 = FALSE  # Visible
              n251 = global read "Meas_global.vi" "Raw data file"() -> (w663:path)
              n252 = Strip Path(path=w663) -> (stripped path=w662:path)  [unwired: 1 out]
              n253 = global write "Calib_global.vi" "Calib Raw Data Folder"(w662) -> ()
              n254 = property on="String" class="Str"("Visible"=w661, "Blinking"=w661) -> ()  [unwired: 2 in, 2 out]
            }
          }
        }
        frame "Refit Curve" {
          # "Another calibration point is not required. Also  checks if there are any points to fit curve to."
        }
      }
      "Status Out" <- w480
    }
    frame #12 {
      n255 = Build Array(w674, w677, w676, w671, w675) -> (w673:dbl[][])
      n256 = call "Sort_Array_Indicies.vi"("unsorted array"=w674) -> ("Sort Index"=w670:i32[])  [unwired: 1 out]
      n257 = for {
        tunnel: w670 -> [w680]
        tunnel: w673 -> [w679] mode=indexing
        tunnel: [w678] -> w672 mode=indexing
        n258 = for {
          tunnel: w680 -> [w683] mode=indexing
          tunnel: w679 -> [w682]
          tunnel: [w681] -> w678 mode=indexing
          n259 = Index Array(array=w682, index=w683) -> (element=w681:dbl)
        }
      }
      "Ref velocity" <- w671
    }
    frame #13 {
      w691 = FALSE  # t/f
      w692 = FALSE  # t/f
      n260 = Index Array(array="Point selector 4", index=0) -> (element=w689:cluster{"Y":dbl, "Y2":dbl, "X":dbl, "t/f":bool})
      n261 = Index Array(array="Point selector 3", index=0) -> (element=w697:cluster{"Y":dbl, "X":dbl, "t/f":bool})
      n262 = Bundle By Name(cluster=w689, "t/f"=w691) -> (w690:cluster{"Y":dbl, "Y2":dbl, "X":dbl, "t/f":bool})
      n263 = Bundle By Name(cluster=w697, "t/f"=w692) -> (w693:cluster{"Y":dbl, "X":dbl, "t/f":bool})
      n264 = Build Array (concatenate)("Point selector 4", w690) -> (w686:T5)
      n265 = Build Array (concatenate)("Point selector 3", w693) -> (w695:cluster{"Y":dbl, "X":dbl, "t/f":bool}[])
      n266 = for {
        tunnel: w695 -> [w713]
        tunnel: w699 -> [w710] mode=indexing
        tunnel: [w712] -> w696 mode=indexing
        tunnel: w686 -> [w711]
        tunnel: [w709] -> w685 mode=indexing
        n267 = Index Array(array=w713, index=w710) -> (element=w712:cluster{"Y":dbl, "X":dbl, "t/f":bool})
        n268 = Index Array(array=w711, index=w710) -> (element=w709:cluster{"Y":dbl, "Y2":dbl, "X":dbl, "t/f":bool})
      }
      n269 = call "Calib_Analyse_fit.vi"("Calib file"=w700, "Input points"=w684, "polynomial order"="polynomial order", "Fixed n"="Fixed n", "n"="n", "Point selector 3"=w696, "Point selector 4"=w685) -> ("Calib const"=→"Calib const":string[][], "Calibration plot"=→"Calibration plot":cluster{cluster{dbl, dbl}[]}[], "Point selector 3 out"=w706:cluster{"Y":dbl, "X":dbl, "t/f":bool}[], "Coefficients"=→"Coefficients":dbl[][], "Point selector 4 out"=w705:T5)  [unwired: 4 out]
      n270 = local write "Point selector 3"(w706) -> ()
      n271 = local write "Point selector 4"(w705) -> ()
    }
    frame #14 {
      w729 = FALSE  # Lock File
      w731 = FALSE  # advisory dialog? (display:T)
      w732 = FALSE  # append to file? (new file:F)
      n272 = global read "Calib_global.vi" "Calib Raw Data Folder"() -> (w722:path)
      n273 = global read "Calib_global.vi" "Calib Raw Data Folder"() -> (w721:path)
      n274 = Strip Path(path=w727) -> (name=w726:string)  [unwired: 1 out]
      n275 = List Folder(path=w722) -> (filenames=w725:string[])  [unwired: 1 in, 5 out]
      n276 = Array Size(array=w725) -> (size(s)=w724:i32)
      n277 = Greater Than 0?(x=w724) -> (x > 0?=w723:bool)
      n278 = Path To String(path=w721) -> (string=w720:string)
      n279 = call "Characters_to_string.vi"("Characters to write"=w720, "Label for characters"="Calib Raw Data Folder") -> ("Output string"=w717:string)
      n280 = Concatenate Strings(w718, w717) -> (w716:string)
      n281 = global read "Calib_global.vi" "Header string"() -> (w730:string)
      n282 = call "Add_label_to_string.vi"("String to write"=w716, "File Label"="Raw data header") -> ("Output string"=w714:string)
      n283 = Concatenate Strings(w730, w714) -> (w728:string)
      n284 = case shown="True" w723 {
        tunnel: w728 -> [_ w736]
        tunnel: w726 -> [_ w735]
        tunnel: w722 -> [_ w733]
        frame False {
        }
        frame True {
          w737 = FALSE  # Lock File
          w738 = FALSE  # append to file? (new file:F)
          w739 = FALSE  # advisory dialog? (display:T)
          n285 = Build Path(base path=w733, name or relative path=w735) -> (appended path=w734:path)
          n286 = call "Write_Characters_To_File.vi"("file path (dialog if empty)"=w734, "advisory dialog? (display:T)"=w739, "character string"=w736, "append to file? (new file:F)"=w738, "Lock File"=w737) -> ()  [unwired: 4 out]
        }
      }
      n287 = call "Write_Characters_To_File.vi"("file path (dialog if empty)"=w727, "advisory dialog? (display:T)"=w731, "character string"=w728, "append to file? (new file:F)"=w732, "Lock File"=w729) -> ()  [unwired: 4 out]
    }
    frame #15 {
      n288 = case shown="\"Take new data point\"" w742 {
        tunnel: w741 -> [w745 _]
        tunnel: w740 -> [w744 _]
        frame "Take new data point" {
          n289 = global read "Calib_global.vi" "Calib Ch No"() -> (w743:i16)
          n290 = stacked-sequence {
            tunnel: w745 -> [w747 w765]
            tunnel: w744 -> [_ w764]
            tunnel: w743 -> [w746 w758]
            frame #0 {
              n291 = Current VI's Path() -> (path=w749:path)
              n292 = call "Running_as_top_level.vi"("Vi path name"=w749) -> ("Top Level"=w748:bool)  [unwired: 1 out]
              n293 = case shown="True" w748 {
                tunnel: w747 -> [_ w752]
                tunnel: w746 -> [_ w750]
                frame False {
                }
                frame True {
                  n294 = call "Measurement.vi"("setup"=Setup."Setup Front Panel", "Post Process"=Post_Process."Take New Data", "File"=Save_Data."Save No Data") -> ()  [unwired: 4 in, 13 out]
                  n295 = Build Array(w752) -> (w753:path[])
                  n296 = Build Array(w750) -> (w754:i16[])
                  n297 = call "Current_Calib_Filenames.vi"("Calib Filename"=w753, "Channel Numbers"=w754, "Mode"=App_Global."Write to Global") -> ()  [unwired: 3 out]
                }
              }
            }
            frame #1 {
              n298 = global read "Calib_global.vi" "Instrument type"() -> (w767:T12)
              n299 = case shown="\"Cross wire velocity\"" w767 {
                tunnel: w758 -> [_ w779 w785]
                tunnel: [path "" ("appended path") w775 w780] -> w766
                tunnel: [FALSE TRUE TRUE] -> w761
                frame "Propeller anemometer", Default {
                }
                frame "Cross wire angle" {
                  n300 = Format Into String(format string="Ch%d_XW_Angle_Calib", w779) -> (resulting string=w774:string)  [unwired: 2 in, 1 out]
                  n301 = call "Setup_Filepath.vi"("Setup File Type"=Setup_Filetype."Calibration Setups", "Filename in"=w774) -> ("Filename Out"=w775:path)  [unwired: 1 out]
                }
                frame "Cross wire velocity" {
                  n302 = Format Into String(format string="Ch%d_XW_Velocity_Calib", w785) -> (resulting string=w781:string)  [unwired: 2 in, 1 out]
                  n303 = call "Setup_Filepath.vi"("Setup File Type"=Setup_Filetype."Calibration Setups", "Filename in"=w781) -> ("Filename Out"=w780:path)  [unwired: 1 out]
                }
              }
              n304 = Array Size(array=w764) -> (size(s)=w763:i32)
              n305 = Greater?(x=w763, y=1) -> (0:w760:bool)
              n306 = And(x=w760, y=w761) -> (x .and. y?=w759:bool)
              n307 = case shown="True" w759 {
                tunnel: w766 -> [_ w770]
                tunnel: w765 -> [_ w769]
                frame False {
                }
                frame True {
                  n308 = call "Copy_with_Check.vi"("Mode"=enum16{"Move", "Copy"}."Copy", "Target Path"=w770, "Variable Target?"=FALSE, "Source Path"=w769) -> ()  [unwired: 1 out]
                }
              }
            }
          }
        }
        frame "Refit Curve" {
        }
      }
    }
    frame #16 {
      n309 = case shown="\"Take a New Calibration Point\"" w786 {
        frame "Show Setup" {
          n310 = local write "Mode"(Calib_mode."Take a New Calibration Point" ("Mode")) -> ()
        }
        frame "Take a New Calibration Point" {
        }
        frame "Refit Curve" {
        }
        frame "Setup Front Panel" {
          n311 = local write "Mode"(Calib_mode."Show Setup" ("Mode")) -> ()
        }
      }
      n312 = global write "Calib_global.vi" "Calibration Points"(dbl[] [] ("Calibration Points")) -> ()
    }
  }
